vi "Close Instrument.vi"(8 "error in (no error)":errorcluster, 11 "Tek 2k Scope.lvclass in":refnum<class "Tek 2k Scope.lvclass">) -> (0 "error out":errorcluster, 3 "Tek 2k Scope.lvclass out":refnum<class "Tek 2k Scope.lvclass">)   [LabVIEW 2010, in "Tek 2k Scope.lvclass"]
uses:
  Tek 2k Scope.lvclass
  Tek 2k Scope.lvclass/Tek 2k Scope.ctl
  <instrlib>/Tektronix TDS 200 1000 2000 Series/Tektronix TDS 200 1000 2000 Series.lvlib
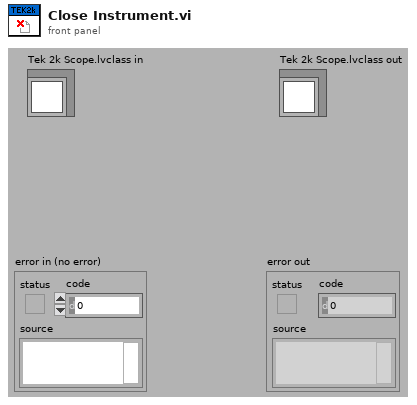
[diagram p1: front panel]
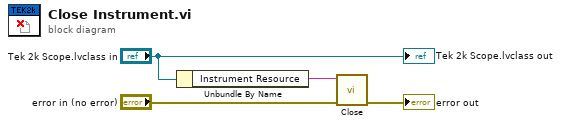
[diagram p0: block diagram]
diagram:
  n1 = Unbundle By Name("Tek 2k Scope.lvclass in") -> ("Instrument Resource"=w1:string)
  n2 = call <instrlib>:"Close.vi"("error in (no error)"="error in (no error)", "VISA resource name"=w1) -> ("error out"=→"error out":errorcluster)  [unwired: 9 out]
  "Tek 2k Scope.lvclass out" <- "Tek 2k Scope.lvclass in"
